vi "Parse Attribute.vi"(4 "Header Values":string[](array[string]), 6 "Header Names":string[](array[string]), 8 "error in (no error)":errorcluster, 9 "Tag Name":string, 10 "Flattened Linked List":string, 11 "XML in":refnum<class "XML.lvclass">) -> (0 "Error Out":errorcluster, 2 "Flattened Linked List out":string, 3 "XML out":refnum<class "XML.lvclass">, 5 "Attribute Value":variant, 7 "Attribute Name":string)   [LabVIEW 2019, in "XML.lvlib" / "XML.lvclass"]
uses:
  <vilib>/gpm_packages/@cs/persistence/source/XML/XML.lvclass
  <vilib>/Utility/error.llb/Error Cluster From Error Code.vi
  <vilib>/ErrorRing/Error Ring.xnode
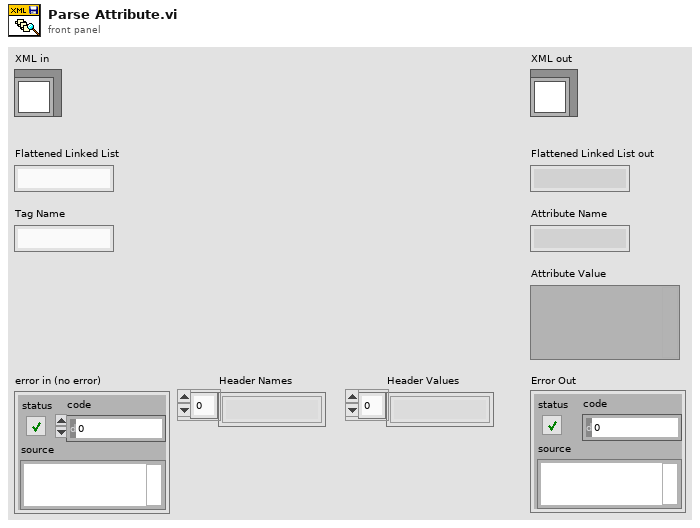
[diagram p1: front panel]
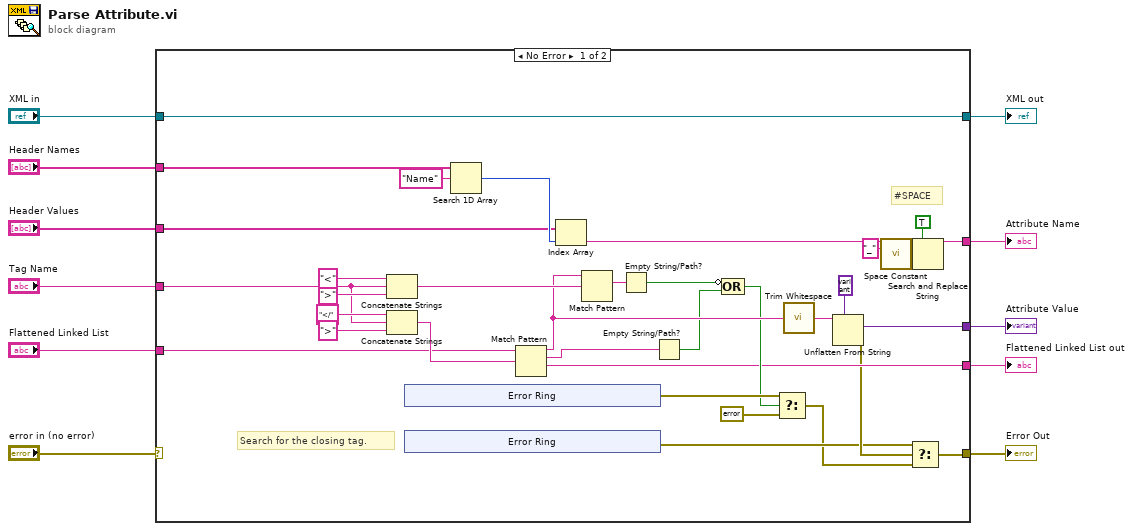
[diagram p0: block diagram]
diagram:
  n1 = case shown="No Error" "error in (no error)" {
    selector: "error in (no error)" -> [_ w56]
    tunnel: "XML in" -> [w22 w58]
    tunnel: "Flattened Linked List" -> [w32 w57]
    tunnel: [w31 w57] -> w9
    tunnel: [w14 _] -> w8
    tunnel: [w28 _] -> w7
    tunnel: [w24 w56] -> w6
    tunnel: [w22 w58] -> w5
    tunnel: "Header Names" -> [w19 _]
    tunnel: "Header Values" -> [w18 _]
    tunnel: "Tag Name" -> [w17 _]
    frame No Error {
      # "#SPACE"
      # "Search for the closing tag."
      n2 = Concatenate Strings("<" ("string"), w17, ">" ("string")) -> (w38:string)
      n3 = Concatenate Strings("</" ("string"), w17, ">" ("string")) -> (w41:string)
      n4 = xnode "Error Ring"() -> ("error out"=w44:errorcluster)
      n5 = xnode "Error Ring"() -> ("error out"=w26:errorcluster)
      n6 = Search 1D Array(1D array=w19, element="Name") -> (index of element=w20:i32)  [unwired: 1 in]
      n7 = Match Pattern(string=w32, regular expression=w41) -> (before substring=w37:string, match substring=w45:string, after substring=w31:string)  [unwired: 1 in, 1 out]
      n8 = Index Array(array=w18, index=w20) -> (element=w15:string)
      n9 = Match Pattern(string=w37, regular expression=w38) -> (match substring=w36:string)  [unwired: 1 in, 3 out]
      n10 = Empty String/Path?(string/path=w36) -> (empty?=w35:bool)
      n11 = Empty String/Path?(string/path=w45) -> (empty?=w34:bool)
      n12 = Compound Arithmetic op=OR(invert w35, w34) -> (w33:bool)
      n13 = Select(t=w44, s=w33, f=errorcluster {"status"=FALSE, "code"=0, "source"=""}) -> (s? t:f=w23:errorcluster)
      n14 = call <vilib>:"Trim Whitespace.vi"("string"=w37) -> ("trimmed string"=w29:string)  [unwired: 1 in]
      n15 = Unflatten From String(type=variant ("variant"), binary string=w29) -> (value=w28:variant, error out=w27:errorcluster)  [unwired: 3 in, 1 out]
      n16 = call <vilib>:"Space Constant.vi"() -> ("String"=w12:string)
      n17 = Select(t=w26, s=w27, f=w23) -> (s? t:f=w24:errorcluster)
      n18 = Search and Replace String(replace all?=TRUE ("replace all? (F)"), input string=w15, search string="_", replace string=w12) -> (result string=w14:string)  [unwired: 4 in, 3 out]
    }
    frame Error {
    }
  }
  "XML out" <- w5
  "Flattened Linked List out" <- w9
  "Attribute Name" <- w8
  "Attribute Value" <- w7
  "Error Out" <- w6
